vi "Init.vi"(8 "error in (no error)":errorcluster, 11 "object in":refnum<class "Board.lvclass">) -> (0 "error out":errorcluster, 3 "object out":refnum<class "Board.lvclass">)   [LabVIEW 2020, in "Board.lvclass"]
doc: "Gets the initial position in FEN notation and places the Pieces in the board, sets the first player to play."
uses:
  Board.lvclass
panel:
  # "This is the FEN of the standard starting position in normal chess\n\nRead this for documentation:\nhttps://en.wikipedia.org/wiki/Forsyth%E2%80%93Edwards_Notation"
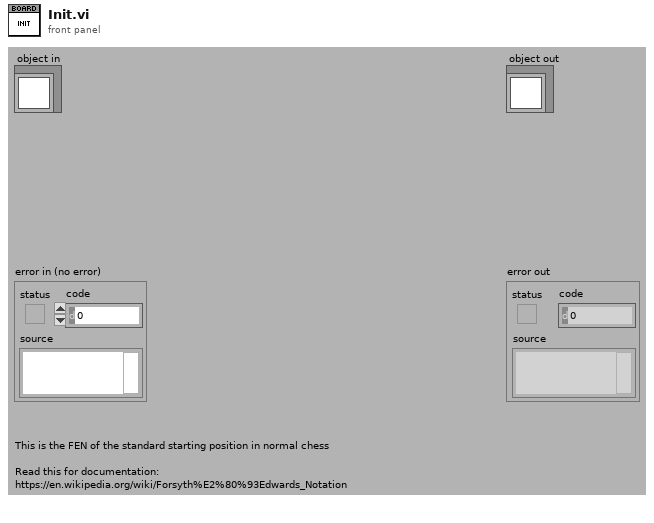
[diagram p1: front panel]
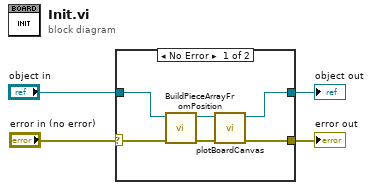
[diagram p0: block diagram]
diagram:
  n1 = case shown="No Error" "error in (no error)" {
    selector: "error in (no error)" -> [w9 w11]
    tunnel: "object in" -> [w10 w12]
    tunnel: [w5 w12] -> w4
    tunnel: [w6 w11] -> w3
    frame No Error {
      n2 = call "BuildPieceArrayFromPosition.vi"("error in (no error)"=w9, "object in"=w10) -> ("error out"=w7:errorcluster, "object out"=w8:refnum<class "Board.lvclass">)  [unwired: 8 in]
      n3 = call "plotBoardCanvas.vi"("error in (no error)"=w7, "object in"=w8) -> ("error out"=w6:errorcluster, "object out"=w5:refnum<class "Board.lvclass">)  [unwired: 8 in]
    }
    frame Error {
    }
  }
  "object out" <- w4
  "error out" <- w3
